vi "OpenEthernetIPConnection.vi"(11 "String":string="192.168.1.10") -> (0 "error out":errorcluster, 3 ".NET Refnum out":refnum<k24>)   [LabVIEW 2022 SP3, in "Motor Controller.lvclass"]
uses:
  Motor Controller.lvclass
  C:/projects/Digilens_IPLC2/Classes/Motor Controller/EEIP.dll
  EEIP.dll
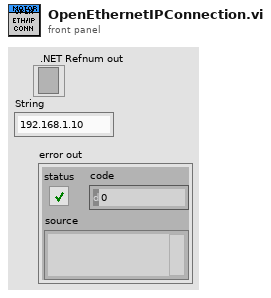
[diagram p1: front panel]
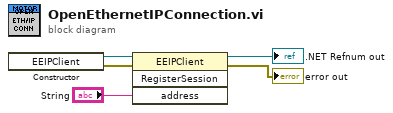
[diagram p0: block diagram]
diagram:
  n1 = constructor class="EEIPClient"() -> (reference out=w1:refnum<k24>, error out=w4:errorcluster)  [unwired: 3 in, 1 out]
  n2 = invoke class="EEIPClient" method="RegisterSession"(reference=w1, error in=w4, "address"="String") -> (reference out=→".NET Refnum out":refnum<k24>, error out=→"error out":errorcluster)  [unwired: 1 in, 2 out]
